vi "Read Item Type.vi"(8 "error in (no error)":errorcluster, 11 "LabVIEWItem in":refnum<class "LabVIEWItem.lvclass">) -> (0 "error out":errorcluster, 2 "VI Type":T1, 3 "LabVIEWItem out":refnum<class "LabVIEWItem.lvclass">)   [LabVIEW 2020, in "Panther Dashboard.lvlib" / "LabVIEWItem.lvclass"]
uses:
  LabVIEWItem.lvclass
  Item Type--enum.ctl
  LabVIEWItem.lvclass/LabVIEWItem.ctl
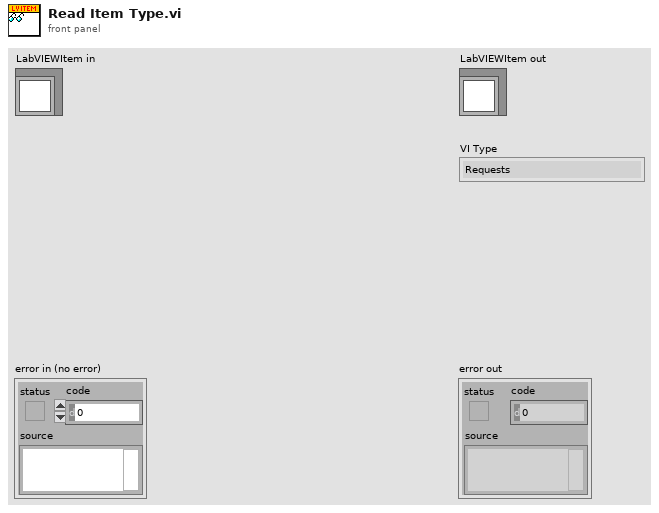
[diagram p1: front panel]
types:
  T1 = typedef "Panther Dashboard.lvlib/LabVIEWItem.lvclass/Item Type--enum.ctl" = enum16{"Requests", "Broadcasts", "Request and Wait for Reply", "Round Trip", "» Public API VIs", "» Constant VIs", "» Error VIs", "Module", "Project", "No Drag Selection"}
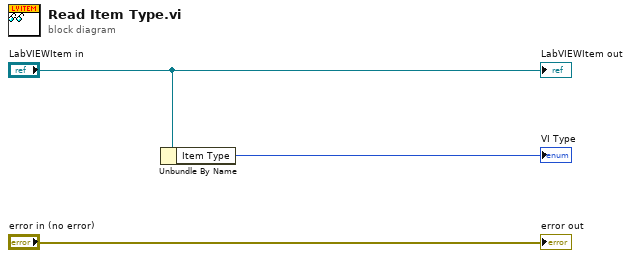
[diagram p0: block diagram]
diagram:
  n1 = Unbundle By Name("LabVIEWItem in") -> ("Item Type"=→"VI Type":T1)
  "error out" <- "error in (no error)"
  "LabVIEWItem out" <- "LabVIEWItem in"
